vi "Save to TDMS.vi"(8 "error in (no error)":errorcluster, 11 "Scan Data Process in":T1) -> (0 "error out":errorcluster, 3 "Scan Data Process out":T1)   [LabVIEW 2015, in "Exposure Process.lvlib"]
uses:
  Exposure Process.lvlib
  Control_Scan Data Process.ctl
  <vilib>/addons/PointValueMap/controls/PointMap.ctl
  Control_EXP Information.ctl
  Control_File Save Setup.ctl
  Control_Enable and Path.ctl
  Control_ICM Export Setting.ctl
  FileHandler/controls/Record.ctl
  FileHandler/FileHandler.lvlib
  <vilib>/addons/PointValueMap/PointValueMap.lvlib
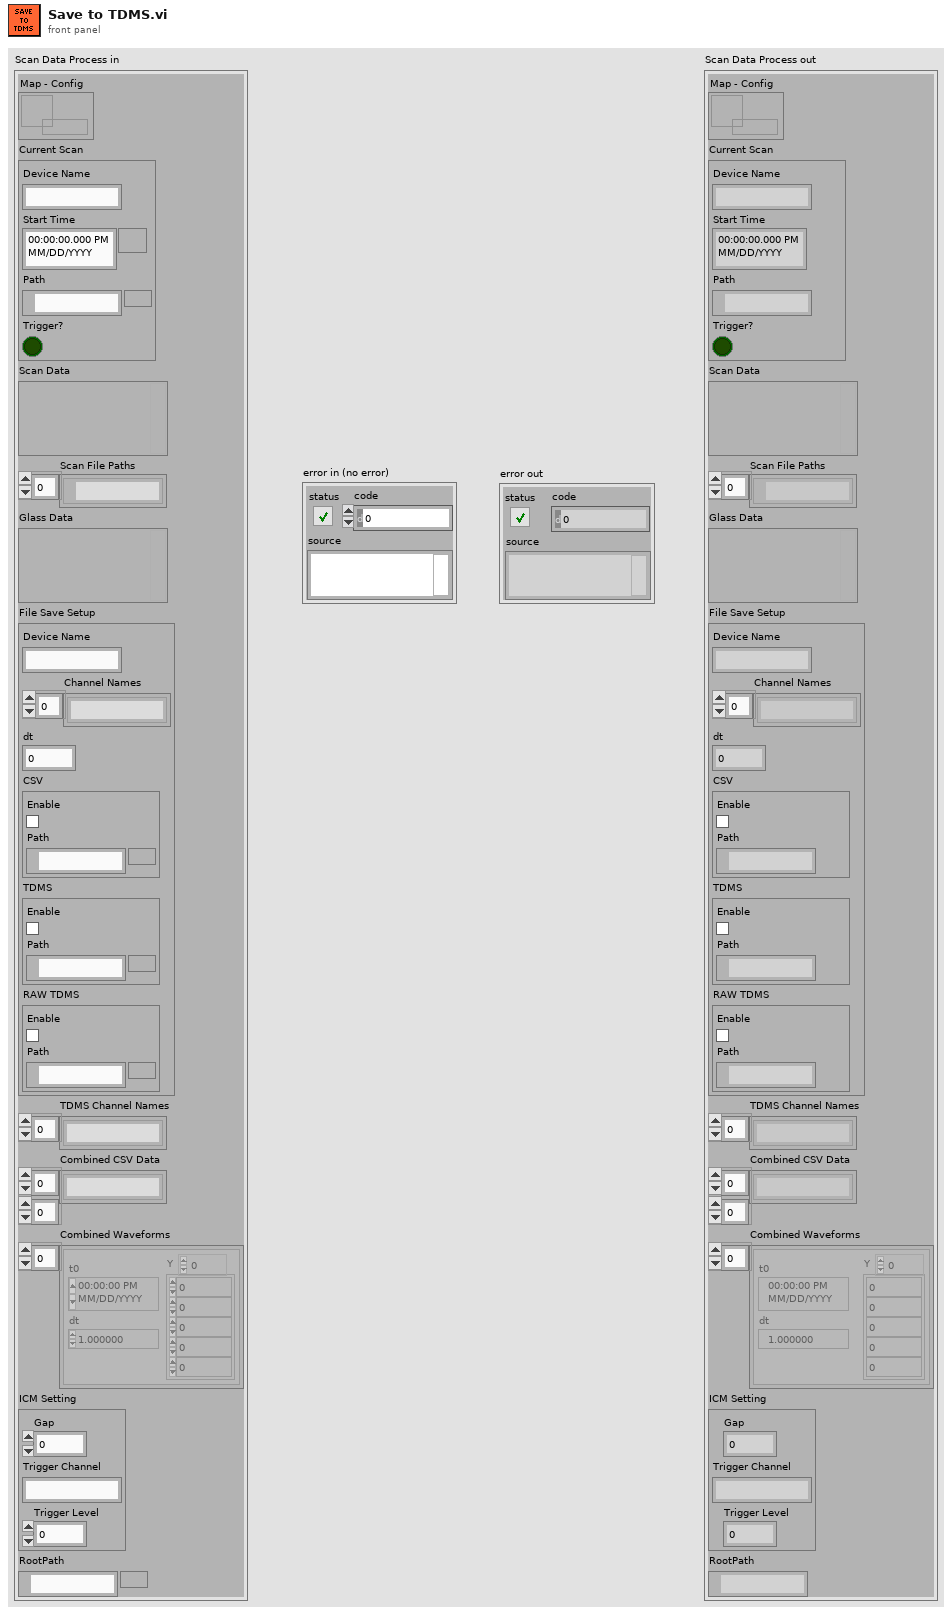
[diagram p1: front panel]
types:
  T1 = typedef "Exposure Process.lvlib/Control_Scan Data Process.ctl" = cluster{"Map - Config":T2, "Current Scan":T3, "Scan Data":variant, "Scan File Paths":path[], "Glass Data":variant, "File Save Setup":T4, "TDMS Channel Names":string[], "Combined CSV Data":string[][], "Combined Waveforms":waveform(dbl)[], "ICM Setting":T6, "RootPath":path}
  T2 = typedef "PointValueMap.lvlib/PointMap.ctl" = refnum<data-value>
  T3 = typedef "Exposure Process.lvlib/Control_EXP Information.ctl" = cluster{"Device Name":string, "Start Time":timestamp, "Path":path, "Trigger?":bool}
  T4 = typedef "Exposure Process.lvlib/Control_File Save Setup.ctl" = cluster{"Device Name":string, "Channel Names":string[], "dt":dbl, "CSV":T5, "TDMS":T5, "RAW TDMS":T5}
  T5 = typedef "Exposure Process.lvlib/Control_Enable and Path.ctl" = cluster{"Enable":bool, "Path":path}
  T6 = typedef "Exposure Process.lvlib/Control_ICM Export Setting.ctl" = cluster{"Gap":dbl, "Trigger Channel":string, "Trigger Level":dbl}
  T7 = typedef "FileHandler.lvlib/Record.ctl" = cluster{"Time":timestamp, "Path":path}
  T8 = enum16{"open", "open or create", "create or replace", "create", "open (read-only)"}
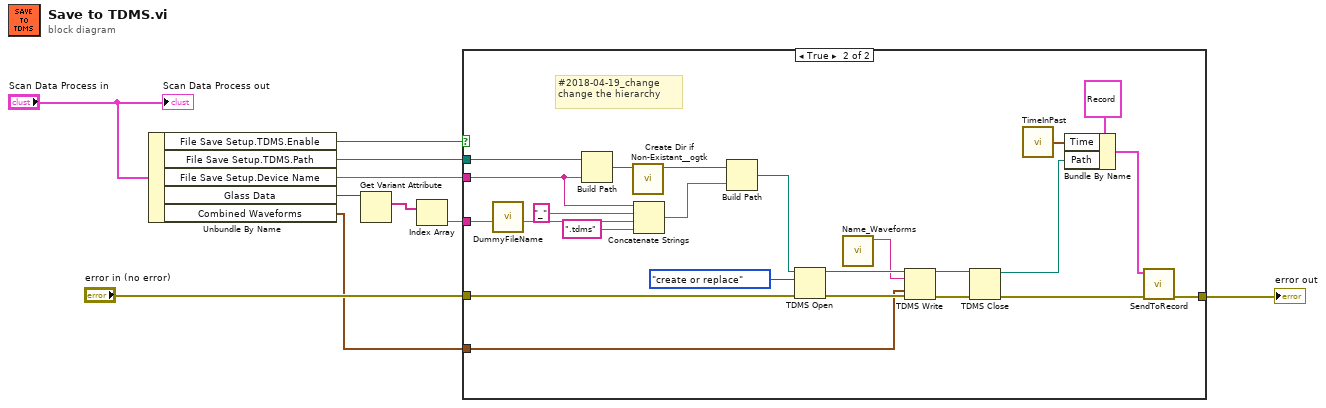
[diagram p0: block diagram]
diagram:
  n1 = Unbundle By Name("Scan Data Process in") -> ("File Save Setup.TDMS.Enable"=w8:bool, "File Save Setup.TDMS.Path"=w7:path, "File Save Setup.Device Name"=w6:string, "Glass Data"=w4:variant, "Combined Waveforms"=w2:waveform(dbl)[])
  n2 = Get Variant Attribute(Variant=w4) -> (names=w5:string[])  [unwired: 3 in, 3 out]
  n3 = Index Array(array=w5) -> (element=w3:string)  [unwired: 1 in]
  n4 = case shown="True" w8 {
    tunnel: "error in (no error)" -> [w11 w30]
    tunnel: [w11 w14] -> w10
    tunnel: w7 -> [_ w20]
    tunnel: w6 -> [_ w19]
    tunnel: w3 -> [_ w24]
    tunnel: w2 -> [_ w23]
    frame False {
    }
    frame True {
      # "#2018-04-19_change\nchange the hierarchy"
      n5 = call "DummyFileName.vi"("Time String in"=w24) -> ("Time String out"=w12:string)  [unwired: 9 in, 1 out]
      n6 = Build Path(base path=w20, name or relative path=w19) -> (appended path=w21:path)
      n7 = call <userlib>:"Create Dir if Non-Existant__ogtk.vi"("Directory Path"=w21) -> ("dup Directory Path"=w22:path)  [unwired: 8 in, 2 out]
      n8 = Concatenate Strings(w19, "_" ("string"), w12, ".tdms" ("string")) -> (w33:string)
      n9 = Build Path(base path=w22, name or relative path=w33) -> (appended path=w32:path)
      n10 = TDMS Open(8:w30, 10:T8."create or replace" ("operation (0:open)"), 11:w32) -> (0:w28:errorcluster, 3:w29:refnum<k34>)  [unwired: 4 in]
      n11 = call "Name_Waveforms.vi"() -> ("Name"=w25:string)  [unwired: 11 in]
      n12 = TDMS Write(0:w29, 5:w25, 9:w23, 11:w28) -> (4:w27:refnum<k34>, 15:w26:errorcluster)  [unwired: 2 in, 2 out]
      n13 = TDMS Close(8:w26, 11:w27) -> (0:w15:errorcluster, 3:w13:path)
      n14 = call "TimeInPast.vi"() -> ("Time Stamp"=w18:timestamp)
      n15 = Bundle By Name(cluster=T7 {"Time"=timestamp(0 s since 1904-01-01), "Path"=path ""} ("Record"), "Time"=w18, "Path"=w13) -> (w17:T7)
      n16 = call "SendToRecord.vi"("error in (no error)"=w15, "Record"=w17) -> ("error out"=w14:errorcluster)  [unwired: 9 in]
    }
  }
  "error out" <- w10
  "Scan Data Process out" <- "Scan Data Process in"
